vi "StrToDBLN.vi"(11 "Array 2":string[](array[string])) -> (0 "Date":string, 3 "number":dbl format="%#_7g")   [LabVIEW 2023]
panel:
  out "output 1":dbl format="%#_7f"
  in  "Zero idx":i32=6
  in  "idx":i32=6
  out "concatenated string":string
  out "element":string
  out "element-1":string
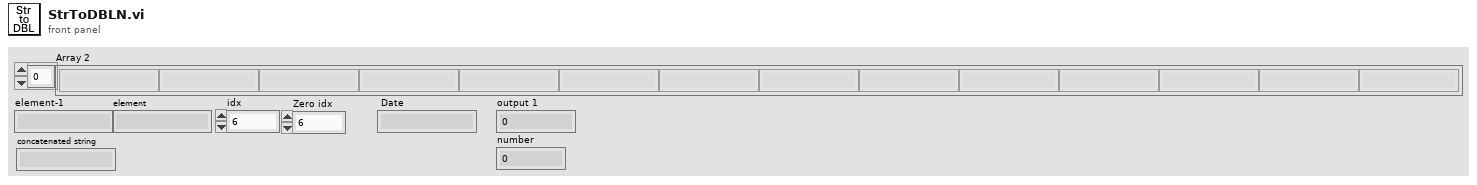
[diagram p1: front panel]
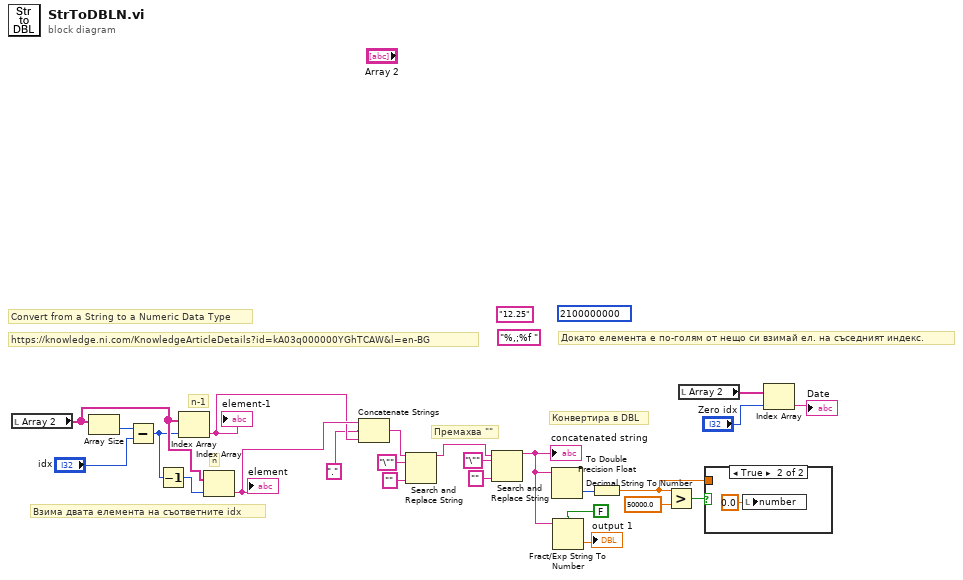
[diagram p0: block diagram]
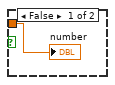
[diagram p2: hidden frame]
diagram:
  (unwired) 2100000000 ("y")
  (unwired) "12.25"
  (unwired) "%,;%f " ("format string")
  # "n"
  # "n-1"
  # "Конвертира в DBL"
  # "Премахва \"\""
  # "Докато елемента е по-голям от нещо си взимай ел. на съседният индекс."
  # "Convert from a String to a Numeric Data Type"
  # "https://knowledge.ni.com/KnowledgeArticleDetails?id=kA03q000000YGhTCAW&l=en-BG"
  # "Взима двата елемента на съответните idx"
  n1 = local read "Array 2"() -> (w19:string[])
  n2 = Array Size(array=w19) -> (size(s)=w21:i32)
  n3 = Subtract(x=w21, y="idx") -> (x-y=w5:i32)
  n4 = Decrement(x=w5) -> (x-1=w20:i32)
  n5 = Index Array(array=w19, index=w5) -> (element=w17:string)
  "element-1" <- w17
  n6 = Index Array(array=w19, index=w20) -> (element=w18:string)
  "element" <- w18
  n7 = Concatenate Strings(w18, "." ("string"), w17) -> (w15:string)
  n8 = Search and Replace String(input string=w15, search string="\"", replace string="" ("replace string (\"\")")) -> (result string=w11:string)  [unwired: 5 in, 3 out]
  n9 = Search and Replace String(input string=w11, search string="\"", replace string="" ("replace string (\"\")")) -> (result string=w7:string)  [unwired: 5 in, 3 out]
  "concatenated string" <- w7
  n10 = Decimal String To Number(string=w7) -> (number=w6:i32)  [unwired: 2 in, 1 out]
  n11 = Fract/Exp String To Number(use system decimal point (T)=FALSE, string=w7) -> (number=→"output 1":dbl)  [unwired: 2 in, 1 out]
  n12 = To Double Precision Float(number=w6) -> (double precision float=w2:dbl)
  n13 = Greater?(x=w2, y=50000.0) -> (0:w3:bool)
  n14 = local read "Array 2"() -> (w24:string[])
  n15 = case shown="True" w3 {
    tunnel: w2 -> [w25 _]
    frame False {
      "number" <- w25
    }
    frame True {
      n16 = local write "number"(0.0 ("number")) -> ()
    }
  }
  n17 = Index Array(array=w24, index="Zero idx") -> (element=→"Date":string)
